vi "setList.vi"(8 "error in (no error)":errorcluster, 10 "list":refnum<class "Shifter.lvclass">[](array[class]), 11 "Shifters in":refnum<class "Shifters.lvclass">) -> (0 "error out":errorcluster, 3 "Shifters out":refnum<class "Shifters.lvclass">)   [LabVIEW 2013, in "Shifters.lvclass"]
uses:
  Shifters.lvclass
  Shifter.lvclass
  Shifters.lvclass/Shifters.ctl
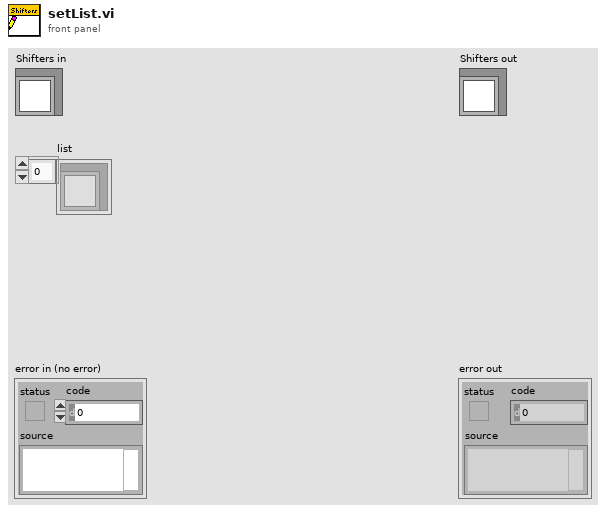
[diagram p1: front panel]
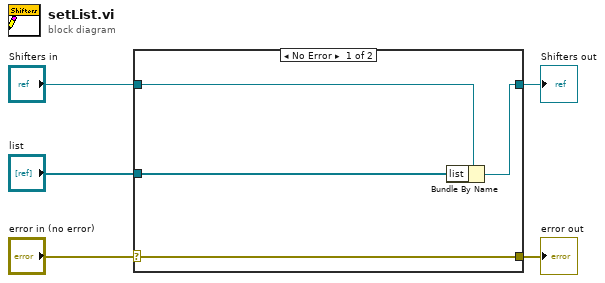
[diagram p0: block diagram]
diagram:
  n1 = case shown="No Error" "error in (no error)" {
    selector: "error in (no error)" -> [w9 w10]
    tunnel: [w9 w10] -> w4
    tunnel: [w7 w11] -> w2
    tunnel: "Shifters in" -> [w8 w11]
    tunnel: "list" -> [w6 _]
    frame No Error {
      n2 = Bundle By Name(cluster=w8, "list"=w6) -> (w7:refnum<class "Shifters.lvclass">)
    }
    frame Error {
    }
  }
  "error out" <- w4
  "Shifters out" <- w2
